vi "GuitarTuner_v2.vi"() -> ()   [LabVIEW 2019]
uses:
  Serial - Settings.ctl
panel:
  in  "String Name":i32=1
  out "Tuner Recommendation":string
  out "String Frequency":dbl format="%.2p"
  out "Measured Soundwave":u16[](graph)
  in  "Stop Time":bool
  in  "Start Time":bool
  in  "VISA resource name":refnum<visa-resource-name>="COM7"
  in  "stop":bool
  # "How to use Guitar Tuner: \n\n1. Set Visa Resource to Correct Channel to Connect to PSoC\n\n2. Click \"Start Time\" to Start the Timer\n\n3. Select String You Want to Tune\n\n4. See Measured String Frequency and Follow Recommendation to Tune the String\n\n5. Click \"Stop Time\" to Stop the Timer\n\n6. Click \"STOP\" to Stop LabVIEW"
  # "String Names:\n1 - E\n2 - A\n3 - D\n4 - G\n5 - B\n6 - E"
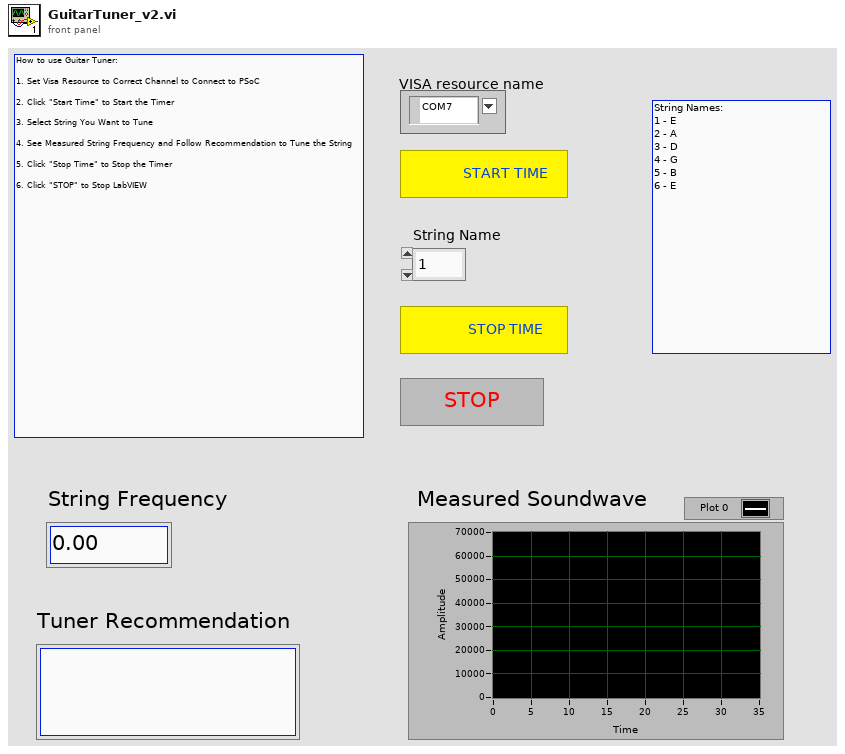
[diagram p1: front panel]
types:
  T1 = typedef "Serial - Settings.ctl" = cluster{"baud rate":u32, "data bits":u16, "parity":enum16{"None", "Odd", "Even", "Mark", "Space"}, "stop bits":u16, "flow control":u16}
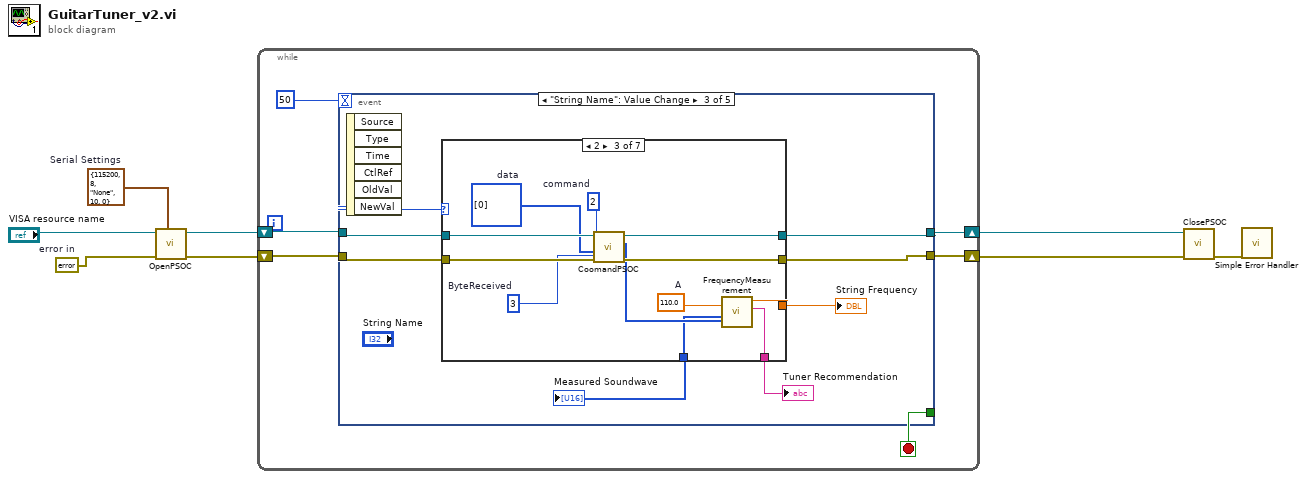
[diagram p0: block diagram]
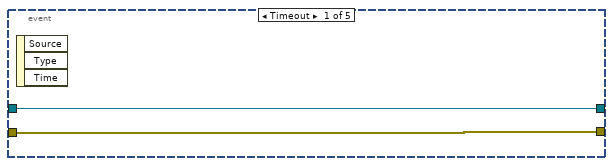
[diagram p2: hidden frame]
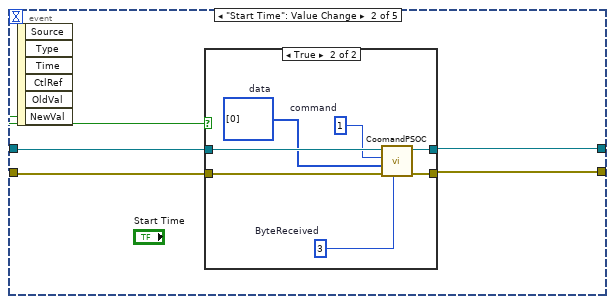
[diagram p3: hidden frame]
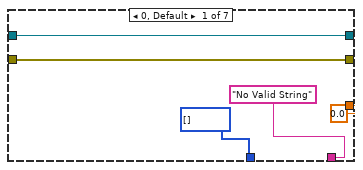
[diagram p5: hidden frame]
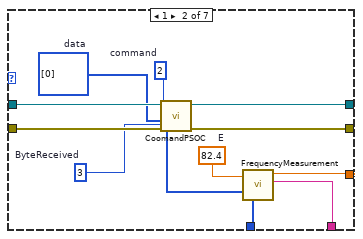
[diagram p6: hidden frame]
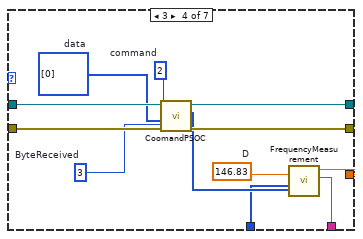
[diagram p7: hidden frame]
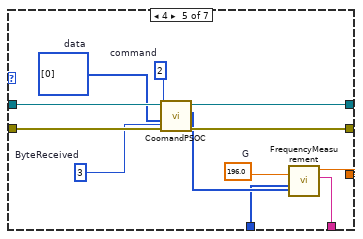
[diagram p8: hidden frame]
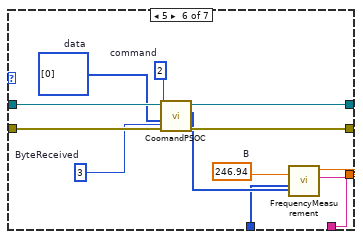
[diagram p9: hidden frame]
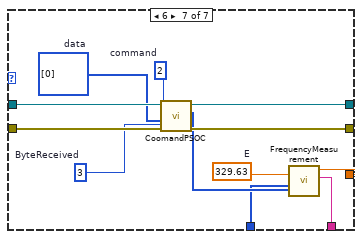
[diagram p10: hidden frame]
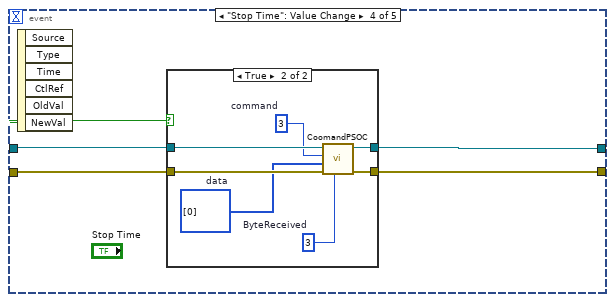
[diagram p11: hidden frame]
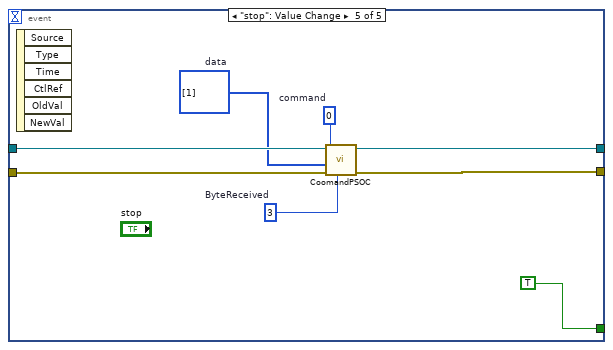
[diagram p13: hidden frame]
diagram:
  w2 = T1 {"baud rate"=115200, "data bits"=8, "parity"=enum."None", "stop bits"=10, "flow control"=0}  # Serial Settings
  w8 = errorcluster {"status"=FALSE, "code"=0, "source"=""}  # error in
  n1 = call "OpenPSOC.vi"("Serial Settings"=w2, "error in"=w8, "VISA resource name"="VISA resource name") -> ("error out"=w6:errorcluster, "VISA resource name out"=w7:refnum<visa-resource-name>)  [unwired: 7 in]
  n2 = while {
    shift-right: [w10] -> w4
    shift-left: w7 -> [w13]
    shift-right: [w11] -> w5
    shift-left: w6 -> [w12]
    stop <- w9 stop-if-true
    n3 = event shown="[2] \"String Name\": Value Change" {
      selector: _ -> [_ _ _ _ _]
      dyn-events: _ -> [_ _ _ _ _]
      timeout: 50 -> [_ _ _ _ _]
      tunnel: w13 -> [w16 w20 w38 w118 w137]
      tunnel: w12 -> [w15 w19 w37 w117 w136]
      tunnel: [w16 w18 w35 w119 w134] -> w10
      tunnel: [w15 w17 w36 w120 w135] -> w11
      tunnel: [_ _ _ _ TRUE] -> w9
      event Timeout {
        n4 = event-data() -> ()  [unwired: 1 in, 3 out]
      }
      event "Start Time": Value Change {
        n5 = event-data() -> ("NewVal"=w21:bool)  [unwired: 1 in, 5 out]
        n6 = case shown="True" w21 {
          tunnel: w20 -> [w23 w30]
          tunnel: w19 -> [w22 w27]
          tunnel: [w22 w29] -> w17
          tunnel: [w23 w28] -> w18
          frame False {
          }
          frame True {
            w24 = u8[] [0]  # data
            w25 = u32 3  # ByteReceived
            w26 = u8 1  # command
            n7 = call "CoomandPSOC.vi"("ByteReceived"=w25, "error in (no error)"=w27, "data"=w24, "command"=w26, "VISA resource name"=w30) -> ("error out"=w29:errorcluster, "VISA resource name out"=w28:refnum<visa-resource-name>)  [unwired: 4 in, 1 out]
          }
        }
      }
      event "String Name": Value Change {
        n8 = event-data() -> ("NewVal"=w34:i32)  [unwired: 1 in, 5 out]
        n9 = case shown="2" w34 {
          tunnel: w38 -> [w43 w55 w67 w79 w91 w103 w115]
          tunnel: w37 -> [w42 w52 w64 w76 w88 w100 w112]
          tunnel: [w42 w54 w66 w78 w90 w102 w114] -> w36
          tunnel: [w43 w53 w65 w77 w89 w101 w113] -> w35
          tunnel: [u16[] [] ("Waveform Graph 2") w46 w58 w70 w82 w94 w106] -> w33
          tunnel: ["No Valid String" ("Tuner Recommendation") w45 w57 w69 w81 w93 w105] -> w32
          tunnel: [0.0 ("detected frequency") w44 w56 w68 w80 w92 w104] -> w31
          frame 0, Default {
          }
          frame 1 {
            w47 = 82.4  # E
            w49 = u8[] [0]  # data
            w50 = u32 3  # ByteReceived
            w51 = u8 2  # command
            n10 = call "CoomandPSOC.vi"("ByteReceived"=w50, "error in (no error)"=w52, "data"=w49, "command"=w51, "VISA resource name"=w55) -> ("error out"=w54:errorcluster, "Command Echo"=w48:u8[], "VISA resource name out"=w53:refnum<visa-resource-name>)  [unwired: 4 in]
            n11 = call "FrequencyMeasurement.vi"("Command Echo"=w48, "Scalar"=w47) -> ("Waveform Graph 2"=w46:u16[], "Tuner Recommendation"=w45:string, "detected frequency"=w44:dbl)  [unwired: 7 in]
          }
          frame 2 {
            w59 = 110.0  # A
            w61 = u8[] [0]  # data
            w62 = u32 3  # ByteReceived
            w63 = u8 2  # command
            n12 = call "CoomandPSOC.vi"("ByteReceived"=w62, "error in (no error)"=w64, "data"=w61, "command"=w63, "VISA resource name"=w67) -> ("error out"=w66:errorcluster, "Command Echo"=w60:u8[], "VISA resource name out"=w65:refnum<visa-resource-name>)  [unwired: 4 in]
            n13 = call "FrequencyMeasurement.vi"("Command Echo"=w60, "Scalar"=w59) -> ("Waveform Graph 2"=w58:u16[], "Tuner Recommendation"=w57:string, "detected frequency"=w56:dbl)  [unwired: 7 in]
          }
          frame 3 {
            w71 = 146.83  # D
            w73 = u8[] [0]  # data
            w74 = u32 3  # ByteReceived
            w75 = u8 2  # command
            n14 = call "CoomandPSOC.vi"("ByteReceived"=w74, "error in (no error)"=w76, "data"=w73, "command"=w75, "VISA resource name"=w79) -> ("error out"=w78:errorcluster, "Command Echo"=w72:u8[], "VISA resource name out"=w77:refnum<visa-resource-name>)  [unwired: 4 in]
            n15 = call "FrequencyMeasurement.vi"("Command Echo"=w72, "Scalar"=w71) -> ("Waveform Graph 2"=w70:u16[], "Tuner Recommendation"=w69:string, "detected frequency"=w68:dbl)  [unwired: 7 in]
          }
          frame 4 {
            w83 = 196.0  # G
            w85 = u8[] [0]  # data
            w86 = u32 3  # ByteReceived
            w87 = u8 2  # command
            n16 = call "CoomandPSOC.vi"("ByteReceived"=w86, "error in (no error)"=w88, "data"=w85, "command"=w87, "VISA resource name"=w91) -> ("error out"=w90:errorcluster, "Command Echo"=w84:u8[], "VISA resource name out"=w89:refnum<visa-resource-name>)  [unwired: 4 in]
            n17 = call "FrequencyMeasurement.vi"("Command Echo"=w84, "Scalar"=w83) -> ("Waveform Graph 2"=w82:u16[], "Tuner Recommendation"=w81:string, "detected frequency"=w80:dbl)  [unwired: 7 in]
          }
          frame 5 {
            w95 = 246.94  # B
            w97 = u8[] [0]  # data
            w98 = u32 3  # ByteReceived
            w99 = u8 2  # command
            n18 = call "CoomandPSOC.vi"("ByteReceived"=w98, "error in (no error)"=w100, "data"=w97, "command"=w99, "VISA resource name"=w103) -> ("error out"=w102:errorcluster, "Command Echo"=w96:u8[], "VISA resource name out"=w101:refnum<visa-resource-name>)  [unwired: 4 in]
            n19 = call "FrequencyMeasurement.vi"("Command Echo"=w96, "Scalar"=w95) -> ("Waveform Graph 2"=w94:u16[], "Tuner Recommendation"=w93:string, "detected frequency"=w92:dbl)  [unwired: 7 in]
          }
          frame 6 {
            w107 = 329.63  # E
            w109 = u8[] [0]  # data
            w110 = u32 3  # ByteReceived
            w111 = u8 2  # command
            n20 = call "CoomandPSOC.vi"("ByteReceived"=w110, "error in (no error)"=w112, "data"=w109, "command"=w111, "VISA resource name"=w115) -> ("error out"=w114:errorcluster, "Command Echo"=w108:u8[], "VISA resource name out"=w113:refnum<visa-resource-name>)  [unwired: 4 in]
            n21 = call "FrequencyMeasurement.vi"("Command Echo"=w108, "Scalar"=w107) -> ("Waveform Graph 2"=w106:u16[], "Tuner Recommendation"=w105:string, "detected frequency"=w104:dbl)  [unwired: 7 in]
          }
        }
        "Measured Soundwave" <- w33
        "Tuner Recommendation" <- w32
        "String Frequency" <- w31
      }
      event "Stop Time": Value Change {
        n22 = event-data() -> ("NewVal"=w116:bool)  [unwired: 1 in, 5 out]
        n23 = case shown="True" w116 {
          tunnel: w118 -> [w122 w129]
          tunnel: w117 -> [w121 w126]
          tunnel: [w121 w128] -> w120
          tunnel: [w122 w127] -> w119
          frame False {
          }
          frame True {
            w123 = u8[] [0]  # data
            w124 = u32 3  # ByteReceived
            w125 = u8 3  # command
            n24 = call "CoomandPSOC.vi"("ByteReceived"=w124, "error in (no error)"=w126, "data"=w123, "command"=w125, "VISA resource name"=w129) -> ("error out"=w128:errorcluster, "VISA resource name out"=w127:refnum<visa-resource-name>)  [unwired: 4 in, 1 out]
          }
        }
      }
      event "stop": Value Change {
        w131 = u32 3  # ByteReceived
        w132 = u8[] [1]  # data
        w133 = u8 0  # command
        n25 = event-data() -> ()  [unwired: 1 in, 6 out]
        n26 = call "CoomandPSOC.vi"("ByteReceived"=w131, "error in (no error)"=w136, "data"=w132, "command"=w133, "VISA resource name"=w137) -> ("error out"=w135:errorcluster, "VISA resource name out"=w134:refnum<visa-resource-name>)  [unwired: 4 in, 1 out]
      }
    }
  }
  n27 = call "ClosePSOC.vi"("error in"=w5, "VISA resource name"=w4) -> ("error out"=w3:errorcluster)  [unwired: 9 in]
  n28 = call <vilib>:"Simple Error Handler.vi"("error in (no error)"=w3) -> ()  [unwired: 4 in, 5 out]
